vi "WriteVXMCfg.vi"(6 "VXM Properties.Serial Port 3":cluster{"Addr":string, "Enable":bool}, 8 "error in (no error)":errorcluster, 9 "VXM Properties.Serial Port":cluster{"Addr":string, "Enable":bool}, 10 "VXM Properties.Serial Port 2":cluster{"Addr":string, "Enable":bool}, 11 "VXMCfg in":refnum<class "VXMCfg.lvclass">) -> (0 "error out":errorcluster, 3 "VXMCfg out":refnum<class "VXMCfg.lvclass">)   [LabVIEW 2018, in "VXMCfg.lvclass"]
uses:
  VXMCfg.lvclass
  VXMCfg.lvclass/VXMCfg.ctl
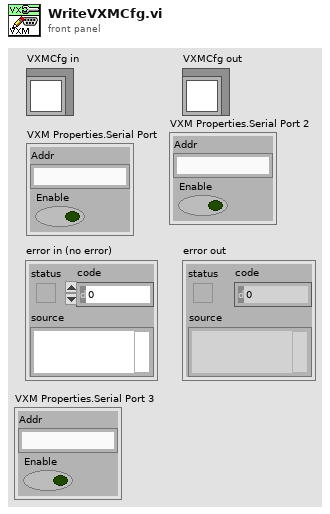
[diagram p1: front panel]
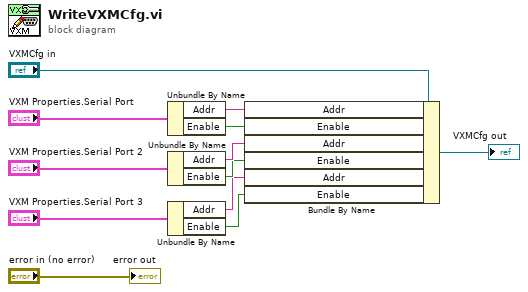
[diagram p0: block diagram]
diagram:
  n1 = Unbundle By Name("VXM Properties.Serial Port") -> ("Addr"=w6:string, "Enable"=w5:bool)
  n2 = Unbundle By Name("VXM Properties.Serial Port 2") -> ("Addr"=w4:string, "Enable"=w3:bool)
  n3 = Unbundle By Name("VXM Properties.Serial Port 3") -> ("Addr"=w2:string, "Enable"=w1:bool)
  n4 = Bundle By Name(cluster="VXMCfg in", "Addr"=w6, "Enable"=w5, "Addr"=w4, "Enable"=w3, "Addr"=w2, "Enable"=w1) -> (→"VXMCfg out":refnum<class "VXMCfg.lvclass">)
  "error out" <- "error in (no error)"
